vi "Read Curve.vi"(4 "Properties":T2 {"Common"."Address" format="%x"}, 6 "LinkData":T15, 8 "Error In":errorcluster, 10 "Link":T16, 11 "WorkspaceManager":T1) -> (0 "Error Out":errorcluster, 1 "NewValue":bool, 2 "TBL1D":cluster{"X":sgl[], "Y":sgl[]}, 3 "WorkspaceManager out":T1)   [LabVIEW 2011]
uses:
  Controls/ECUMC Item.ctl
  Controls/LinkData.ctl
  <vilib>/ECUMC/NIVS/Support Files.llb/Item Properties.ctl
  <vilib>/ECUMC/NIVS/Support Files.llb/Address Property.ctl
  <vilib>/ECUMC/NIVS/Support Files.llb/Extension Property.ctl
  <vilib>/ECUMC/NIVS/Support Files.llb/Data Type Property.ctl
  <vilib>/ECUMC/NIVS/Support Files.llb/Byte Order Property.ctl
  <vilib>/ECUMC/NIVS/Support Files.llb/Maximum Property.ctl
  <vilib>/ECUMC/NIVS/Support Files.llb/Minimum Property.ctl
  <vilib>/ECUMC/NIVS/Support Files.llb/Read Only Property.ctl
  <vilib>/ECUMC/NIVS/Support Files.llb/Unit Property.ctl
  <vilib>/ECUMC/NIVS/Support Files.llb/Comment Property.ctl
  <vilib>/ECUMC/NIVS/Support Files.llb/X Dimension Property.ctl
  <vilib>/ECUMC/NIVS/Support Files.llb/Y Dimension Property.ctl
  <vilib>/ECUMC/NIVS/Support Files.llb/Is Virtual Property.ctl
  <vilib>/NI Veristand/Execution/Workspace/WorkspaceAPI.ctl
  NationalInstruments.VeriStand.ClientAPI
  <vilib>/ECUMC/NIVS/Support Files.llb/Get Single Char Data (TCP).vi
  <vilib>/NI Veristand/Execution/Workspace/NI VeriStand - Get Multiple Channel Values.vi
  <vilib>/ECUMC/NIVS/XCPCCP Add-On Execution API.lvlib
  <vilib>/NI Veristand/Execution/Workspace/NI_VS Workspace ExecutionAPI.lvlib
  <vilib>/ECUMC/NIVS/Support Files.llb/XCP and CCP Master Custom Device.lvlib
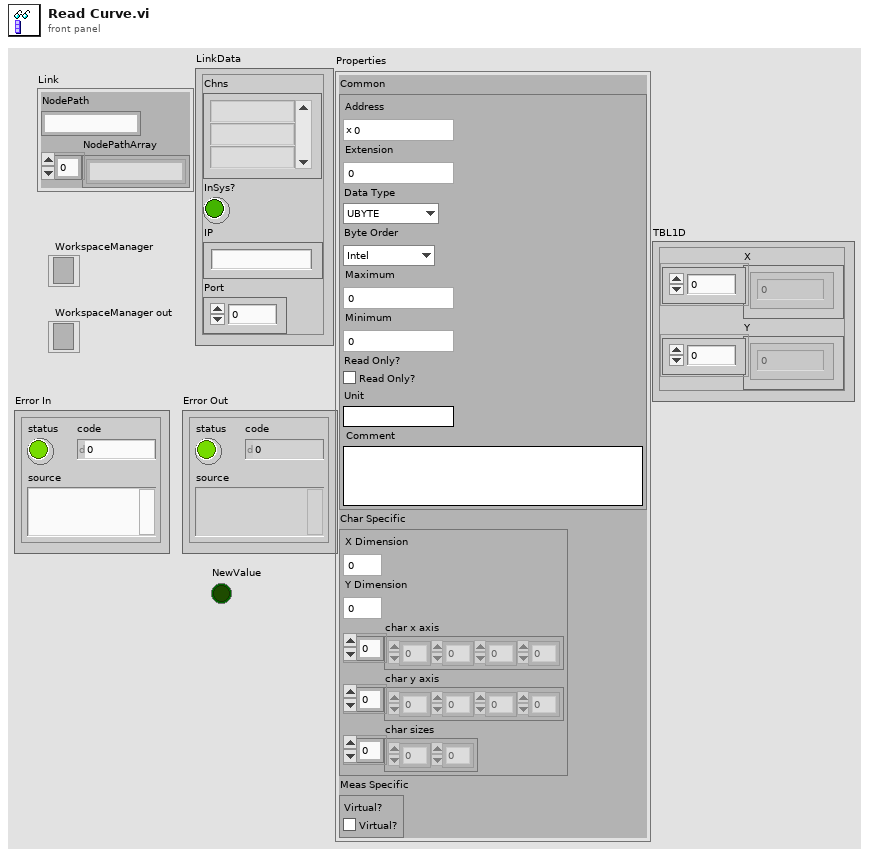
[diagram p1: front panel]
types:
  T1 = typedef "NI_VS Workspace ExecutionAPI.lvlib/WorkspaceAPI.ctl" = refnum<k24>
  T2 = typedef "XCP and CCP Master Custom Device.lvlib/Item Properties.ctl" = cluster{"Common":cluster{"Address":T3, "Extension":T4, "Data Type":T5, "Byte Order":T6, "Maximum":T7, "Minimum":T8, "Read Only?":T9, "Unit":T10, "Comment":T11}, "Char Specific":cluster{"X Dimension":T12, "Y Dimension":T13, "char x axis":dbl[], "char y axis":dbl[], "char sizes":u32[]}, "Meas Specific":cluster{"Virtual?":T14}}
  T3 = typedef "XCP and CCP Master Custom Device.lvlib/Address Property.ctl" = u32
  T4 = typedef "XCP and CCP Master Custom Device.lvlib/Extension Property.ctl" = u8
  T5 = typedef "XCP and CCP Master Custom Device.lvlib/Data Type Property.ctl" = enum16{"UBYTE", "SBYTE", "UWORD", "SWORD", "ULONG", "SLONG", "FLOAT32_IEEE", "FLOAT64_IEEE"}
  T6 = typedef "XCP and CCP Master Custom Device.lvlib/Byte Order Property.ctl" = enum16{"Intel", "Motorola"}
  T7 = typedef "XCP and CCP Master Custom Device.lvlib/Maximum Property.ctl" = dbl
  T8 = typedef "XCP and CCP Master Custom Device.lvlib/Minimum Property.ctl" = dbl
  T9 = typedef "XCP and CCP Master Custom Device.lvlib/Read Only Property.ctl" = bool
  T10 = typedef "XCP and CCP Master Custom Device.lvlib/Unit Property.ctl" = string
  T11 = typedef "XCP and CCP Master Custom Device.lvlib/Comment Property.ctl" = string
  T12 = typedef "XCP and CCP Master Custom Device.lvlib/X Dimension Property.ctl" = u32
  T13 = typedef "XCP and CCP Master Custom Device.lvlib/Y Dimension Property.ctl" = u32
  T14 = typedef "XCP and CCP Master Custom Device.lvlib/Is Virtual Property.ctl" = bool
  T15 = typedef "LinkData.ctl" = cluster{"Chns":string[], "InSys?":bool, "IP":string, "Port":u16}
  T16 = typedef "ECUMC Item.ctl" = cluster{"NodePath":string, "NodePathArray":string[]}
  T17 = typedef "XCP and CCP Master Custom Device.lvlib/Char Data (TCP).ctl" = cluster{"1d":dbl[], "2d":dbl[][], "Single":dbl, "Size":T18}
  T18 = typedef "XCP and CCP Master Custom Device.lvlib/Char Size for TCP.ctl" = enum16{"Single", "1d", "2d"}
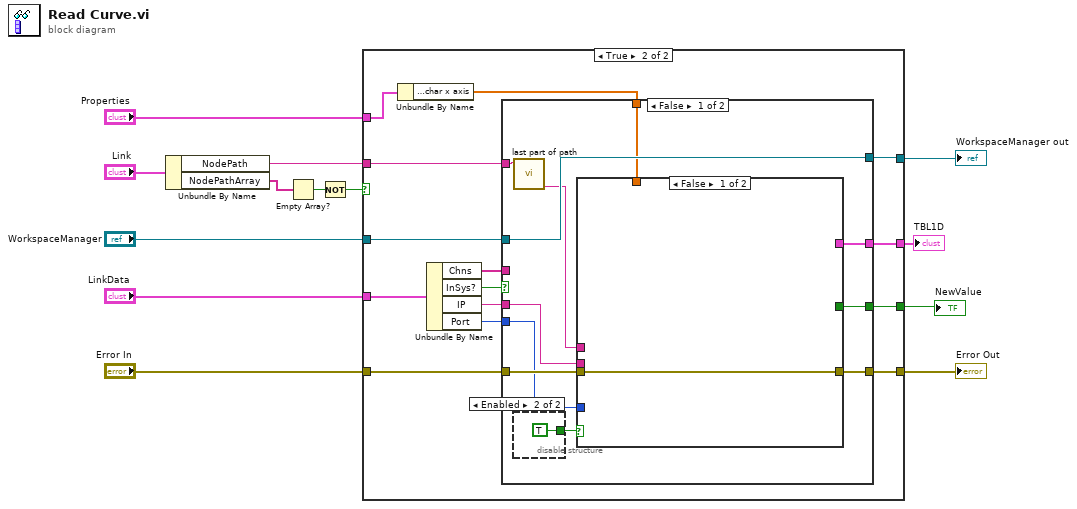
[diagram p0: block diagram]
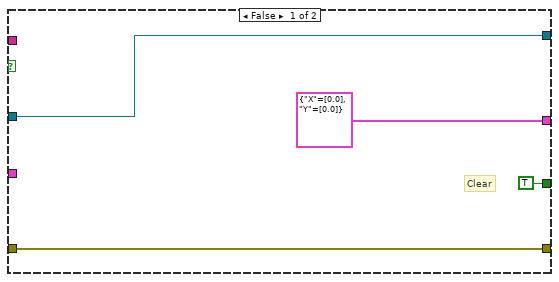
[diagram p2: hidden frame]
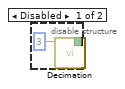
[diagram p3: hidden frame]
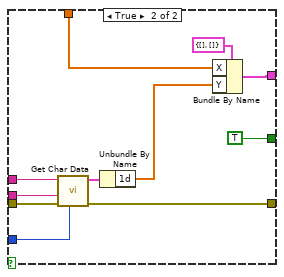
[diagram p4: hidden frame]
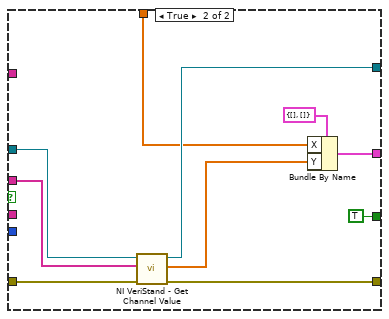
[diagram p5: hidden frame]
diagram:
  n1 = Unbundle By Name("Link") -> ("NodePath"=w10:string, "NodePathArray"=w6:string[])
  n2 = Empty Array?(array=w6) -> (empty?=w4:bool)
  n3 = Not(x=w4) -> (.not. x?=w3:bool)
  n4 = case shown="True" w3 {
    tunnel: "LinkData" -> [_ w31]
    tunnel: "Error In" -> [w17 w28]
    tunnel: w10 -> [_ w20]
    tunnel: "Properties" -> [_ w19]
    tunnel: [cluster{"X":sgl[], "Y":sgl[]} {"X"=[0.0], "Y"=[0.0]} ("TBL1D") w21] -> w2
    tunnel: "WorkspaceManager" -> [w16 w25]
    tunnel: [w17 w24] -> w7
    tunnel: [w16 w23] -> w5
    tunnel: [TRUE w18] -> w1
    frame False {
      # "Clear"
    }
    frame True {
      n5 = Unbundle By Name(w19) -> ("Char Specific.char x axis"=w22:dbl[])
      n6 = Unbundle By Name(w31) -> ("Chns"=w29:string[], "InSys?"=w30:bool, "IP"=w27:string, "Port"=w26:u16)
      n7 = case shown="False" w30 {
        tunnel: w29 -> [_ w67]
        tunnel: w25 -> [w38 w66]
        tunnel: w28 -> [w42 w65]
        tunnel: [w41 w64] -> w24
        tunnel: w27 -> [w40 _]
        tunnel: w26 -> [w39 _]
        tunnel: [w38 w63] -> w23
        tunnel: w22 -> [w36 w61]
        tunnel: [w35 w62] -> w21
        tunnel: w20 -> [w34 _]
        tunnel: [w32 TRUE] -> w18
        frame False {
          n8 = call "last part of path.vi"("String"=w34) -> ("Last Part"=w33:string)  [unwired: 10 in]
          n9 = disable-structure shown="Enabled" {
            disable-tunnel: [w43 TRUE ("Trigger")] -> w37
            frame Disabled {
              n10 = call "Decimation.vi"("Decimation Factor"=3) -> ("Trigger"=w43:bool)  [unwired: 10 in]
            }
            frame Enabled {
            }
          }
          n11 = case shown="False" w37 {
            tunnel: w42 -> [w46 w57]
            tunnel: [w46 w56] -> w41
            tunnel: w40 -> [_ w55]
            tunnel: w39 -> [_ w54]
            tunnel: w33 -> [_ w52]
            tunnel: w36 -> [_ w49]
            tunnel: [_ w50] -> w35
            tunnel: [_ TRUE] -> w32
            frame False {
            }
            frame True {
              n12 = call-poly <vilib>:"Get Char Data.vi"("Port"=w54, "error in (no error)"=w57, "IP or DNS Name"=w55, "Characteristic"=w52) -> ("error out"=w56:errorcluster, "Characteristic Data"=w53:T17)  [unwired: 6 in]
              n13 = Unbundle By Name(w53) -> ("1d"=w51:dbl[])
              n14 = Bundle By Name(cluster=cluster{"X":sgl[], "Y":sgl[]} {"X"=[], "Y"=[]} ("TBL1D"), "X"=w49, "Y"=w51) -> (w50:cluster{"X":sgl[], "Y":sgl[]})
            }
          }
        }
        frame True {
          n15 = call-poly <vilib>:"NI VeriStand - Get Channel Value.vi"("error in (no error)"=w65, "Channels"=w67, "WorkspaceManager in"=w66) -> ("error out"=w64:errorcluster, "Values"=w60:dbl[], "WorkspaceManager out"=w63:T1)  [unwired: 6 in]
          n16 = Bundle By Name(cluster=cluster{"X":sgl[], "Y":sgl[]} {"X"=[], "Y"=[]} ("TBL1D"), "X"=w61, "Y"=w60) -> (w62:cluster{"X":sgl[], "Y":sgl[]})
        }
      }
    }
  }
  "Error Out" <- w7
  "WorkspaceManager out" <- w5
  "TBL1D" <- w2
  "NewValue" <- w1
